vi "INI-RWtabs-EnFlo.vi"(6 "Mode":enum16{"Read", "Write"}(ring), 7 "prompt":string="Please select or create config file", 9 "tabPagesReference":refnum<vi>[](array[refnum]), 11 "INIfilepathIn":path) -> (3 "INIfilepathOut":path)   [LabVIEW 2021]
uses:
  <vilib>/Utility/config.llb/NI_LVConfig.lvlib
panel:
  # "Makes best effort attempt to save/ restore values of all controls on multiple tabs to an INI file"
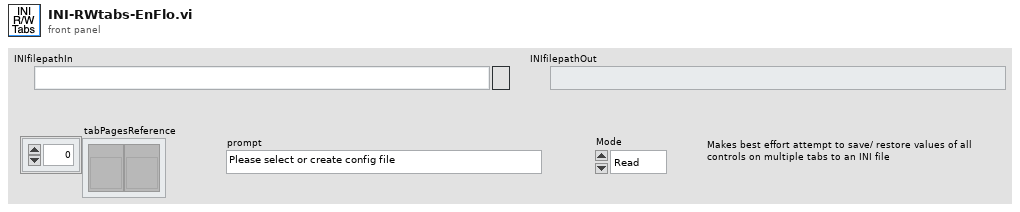
[diagram p1: front panel]
types:
  T1 = typedef "NI_LVConfig.lvlib/Config Data RefNum.ctl" = refnum<k1>
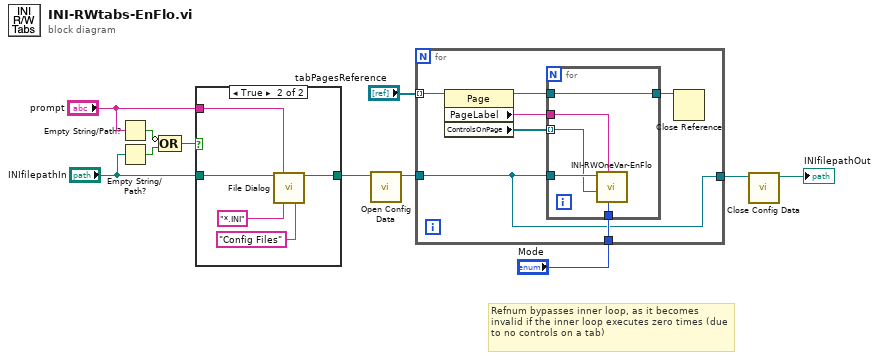
[diagram p0: block diagram]
diagram:
  # "Refnum bypasses inner loop, as it becomes invalid if the inner loop executes zero times (due to no controls on a tab)"
  n1 = Empty String/Path?(string/path="prompt") -> (empty?=w3:bool)
  n2 = Empty String/Path?(string/path="INIfilepathIn") -> (empty?=w2:bool)
  n3 = Compound Arithmetic op=OR(invert w3, w2) -> (w1:bool)
  n4 = case shown="True" w1 {
    tunnel: "INIfilepathIn" -> [w12 w14]
    tunnel: [w12 w17] -> w8
    tunnel: "prompt" -> [_ w13]
    frame False {
    }
    frame True {
      n5 = call "File Dialog"("start path"=w14, "prompt"=w13, "pattern (all files)"="*.INI", "pattern label"="Config Files") -> ("selected path"=w17:path)  [unwired: 8 in, 3 out]
    }
  }
  n6 = call <vilib>:"Open Config Data.vi"("configuration file path"=w8) -> ("refnum"=w11:T1)  [unwired: 8 in, 2 out]
  n7 = for {
    tunnel: "tabPagesReference" -> [w23] mode=indexing
    tunnel: w11 -> [w18]
    tunnel: [w18] -> w7
    tunnel: "Mode" -> [w19]
    n8 = property class="Page"(reference=w23) -> (reference out=w21:refnum<vi>, "PageLabel"=w22:string, "ControlsOnPage"=w24:refnum<vi>[])  [unwired: 1 in, 1 out]
    n9 = for {
      tunnel: w24 -> [w27] mode=indexing
      tunnel: w18 -> [w29]
      tunnel: w22 -> [w28]
      tunnel: [w26] -> w20
      tunnel: w21 -> [w26]
      tunnel: w19 -> [w25]
      n10 = call "INI-RWOneVar-EnFlo.vi"("Mode"=w25, "section"=w28, "controlRefIn"=w27, "INIfileRefIn"=w29) -> ()  [unwired: 7 in, 1 out]
    }
    n11 = Close Reference(reference=w20) -> ()  [unwired: 1 in, 1 out]
  }
  n12 = call <vilib>:"Close Config Data.vi"("refnum"=w7) -> ("file path"=→"INIfilepathOut":path)  [unwired: 9 in, 1 out]
